vi "Destory_User_Event.vi"(8 "error in (no error)":errorcluster, 11 "user event In":refnum<user-event>) -> (0 "error out":errorcluster)   [LabVIEW 2014, in "User_Event_Library.lvlib"]
uses:
  User_Event_Library.lvlib
  TypeDef.ctl
panel:
  # "設定User_Event_In為必接"
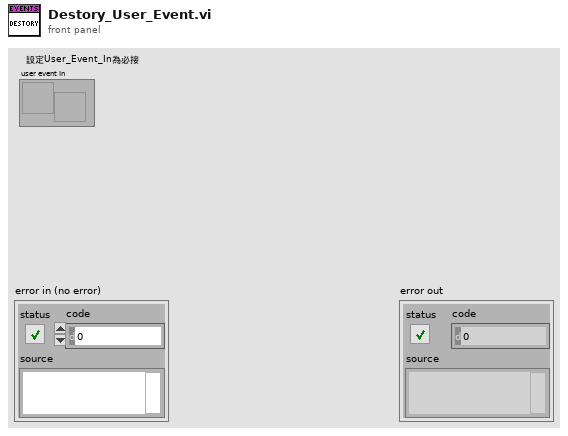
[diagram p1: front panel]
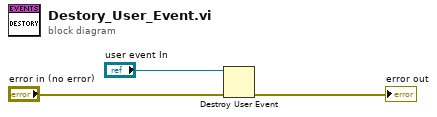
[diagram p0: block diagram]
diagram:
  n1 = Destroy User Event(user event="user event In", error in="error in (no error)") -> (error out=→"error out":errorcluster)
